vi "CheckPortsArray.vi"(2 "INP Ports Array 2":cluster{"String":string, "Array 2":bool[]}[](array[cluster]), 3 "INP":refnum<vi>) -> (0 "Value":i8[](array[numeric]), 1 "INP Ports Array":cluster{"String":string, "Array 2":bool[]}[](array[cluster]))   [LabVIEW 2010]
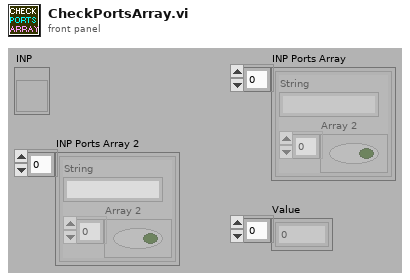
[diagram p1: front panel]
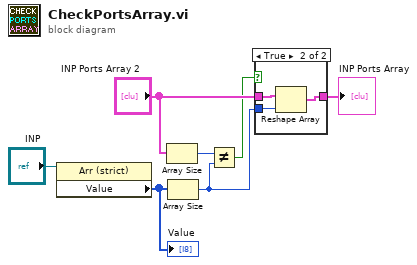
[diagram p0: block diagram]
diagram:
  n1 = property class="Arr (strict)"(reference="INP") -> ("Value"=w3:i8[])  [unwired: 1 in, 2 out]
  "Value" <- w3
  n2 = Array Size(array="INP Ports Array 2") -> (size(s)=w2:i32)
  n3 = Array Size(array=w3) -> (size(s)=w6:i32)
  n4 = Not Equal?(x=w2, y=w6) -> (x != y?=w4:bool)
  n5 = case shown="True" w4 {
    tunnel: "INP Ports Array 2" -> [w8 w11]
    tunnel: w6 -> [_ w10]
    tunnel: [w8 w9] -> w7
    frame False {
    }
    frame True {
      n6 = Reshape Array(w11, w10) -> (w9:cluster{"String":string, "Array 2":bool[]}[])
    }
  }
  "INP Ports Array" <- w7
